vi "TAT_Start_old.vi"(8 "error In":errorcluster) -> (0 "error out":errorcluster)   [LabVIEW 2017]
uses:
  Controls/Ass. Loop Control.ctl
  <vilib>/addons/database/NI_Database_API.lvlib
  <vilib>/addons/database/Connection.llb/DB Tools Open Connec (Path).vi
  <vilib>/Instr/_visa.llb/VISA Configure Serial Port (Instr).vi
  <vilib>/addons/database/Connection.llb/Conn ObjectReference.ctl
  <vilib>/Utility/error.llb/DialogType.ctl
panel:
  out "BARCODE STATION 3":string caption="BARCODE:-"
  out "LEAK UNIT RESULT 2":bool caption="LEAK RESULT:-"
  out "LEAK ACTUAL VALUE 2":string
  out "LEAK MAX 2":string
  out "LEAK MIN 2":string
  out "LEAK UNIT RESULT":bool caption="LEAK RESULT:-"
  out "LEAK ACTUAL VALUE":string
  out "LEAK MAX":string
  out "LEAK MIN":string
  out "PREVIOUS BARCODE":string[](array[string])
  out "scanned":string
  out "PACKAGE Qty  2":string
  out "PROJECT :-":string
  out "PACKAGE Qty":string
  out "TORISHI CODE:-":string
  out "PART No.:-":string
  out "PLC COMMUNICATION":bool
  in  "Stop":bool
  out "BARCODE STATION 2":string caption="BARCODE:-"
  out "RESULT STATION 1":bool caption="FINAL RESULT:-"
  out "USER:-":string
  out "PART NAME :-":string
  in  "ASS-Alarms":bool
  out "CYCLE STATUS STATION 1":string caption="CYCLE STATUS:-"
  out "DATE/TIME":string
  # "KAPSE SONS ROBOTICS\n& AUTOMATION"
  # "PACKAGING SLIP"
  # "MODEL SELECTED"
  # "SCANNED QUANTITY"
  # "PACKAGE QUANTITY"
  # "LEAK TESTING PARAMETER"
  # "MIN"
  # "MAX"
  # "ACTUAL VALUE"
  # "RESULT"
  # "LEAK UNIT"
  # "LEAK PRESSURE"
  # "PREVIOUS BARCODE"
  # "Nm"
  # "POKA-YOKE STATUS"
  # "XBA ORVM"
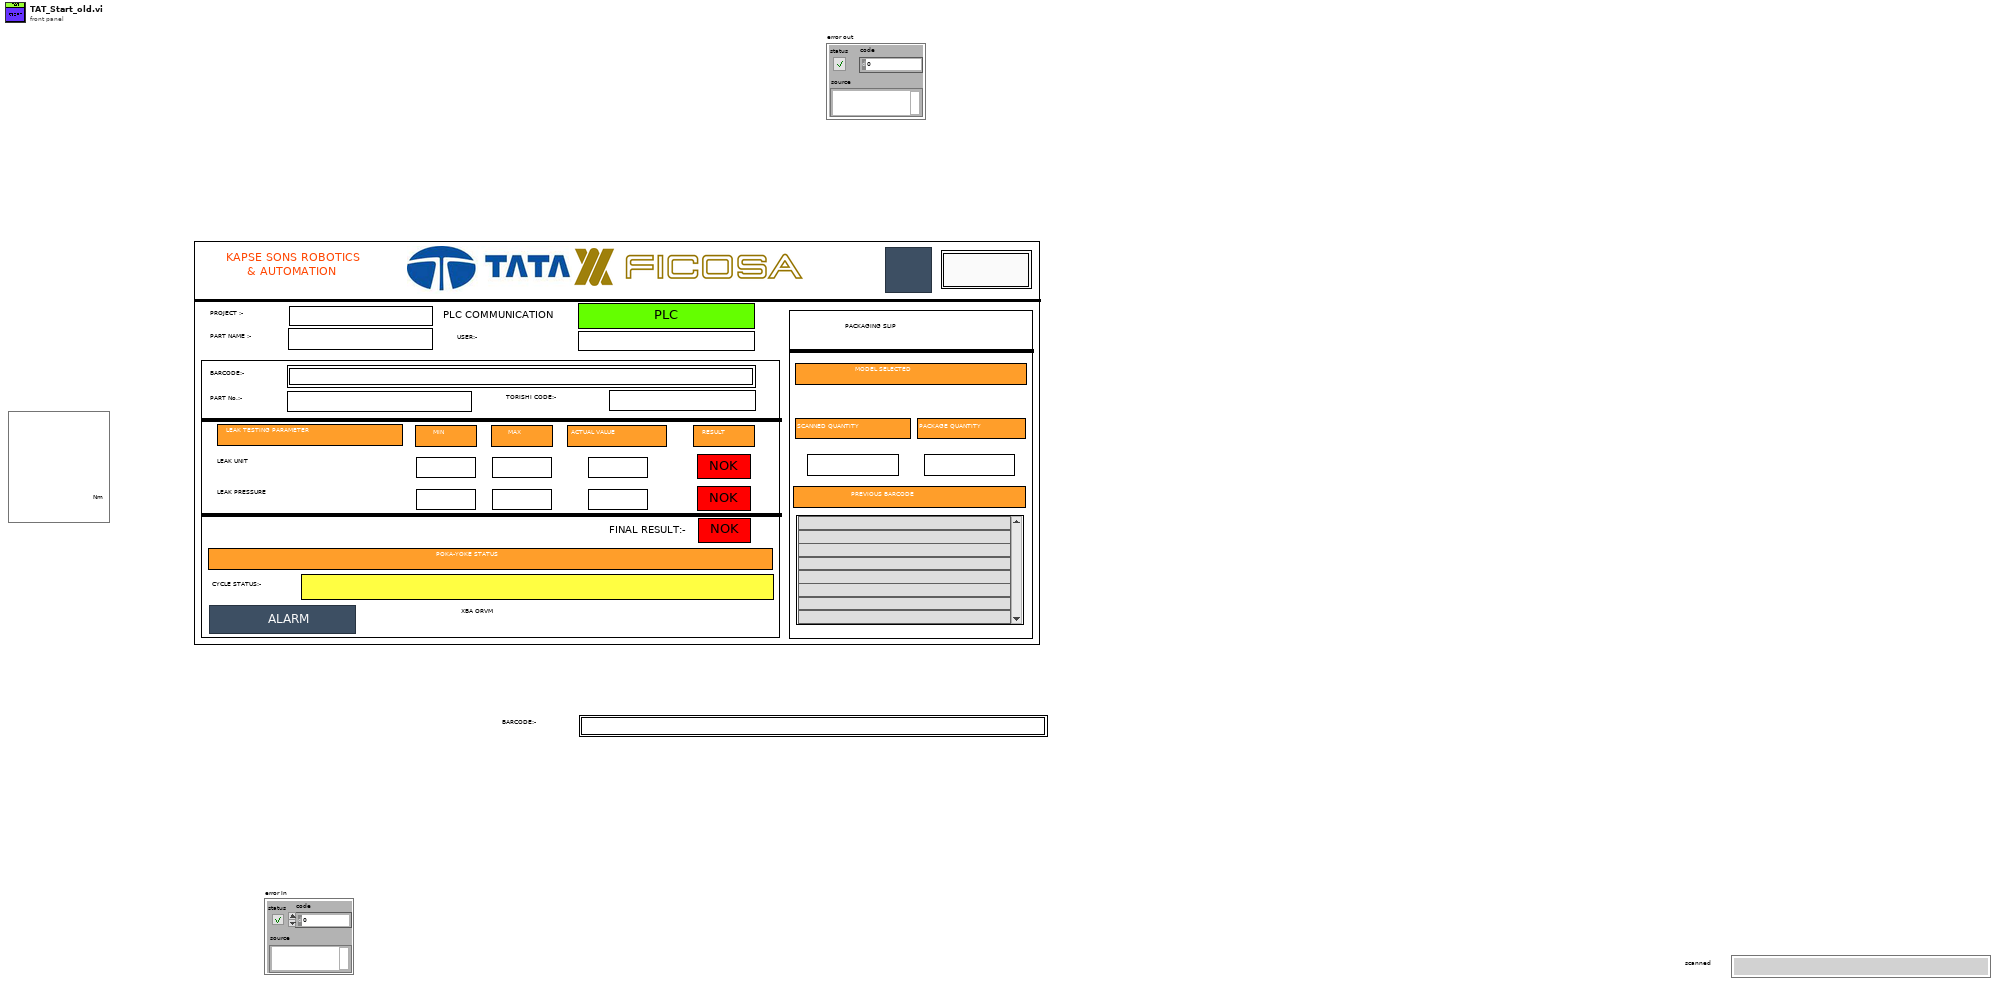
[diagram p1: front panel]
types:
  T1 = typedef "Ass. Loop Control.ctl" = enum16{"Package_Qty_Count", "GENERATE_QR_PRNT", "Cluster_update", "Waiting_for_scan", "barcode CHECK", "Int", "SaveReport ", "Barcode Print", "Start Cycle", "Wait", "Cycle End", "Stop"}
  T2 = typedef "DialogType.ctl" = u16
  T3 = typedef "NI_Database_API.lvlib/Conn ObjectReference.ctl" = refnum<k1>
  T4 = cluster{"Varient number":u16, "Part name":string, "Barcode":string, "connection reference":T3, "Batch_Size":u16, "PART_NO":string, "TORISHI_CODE":string, "printer com":refnum<visa-resource-name>, "scanner com":refnum<visa-resource-name>}
  T5 = cluster{"seconds since 1Jan1904":timestamp, "Part name":string, "BARCODE STATION 2":string, "table":string, "table":string}
  T6 = cluster{"date string":string, "time string":string, "Part name":string, "PART_NO":string, "TORISHI_CODE":string, "table":string, "table":string, string}
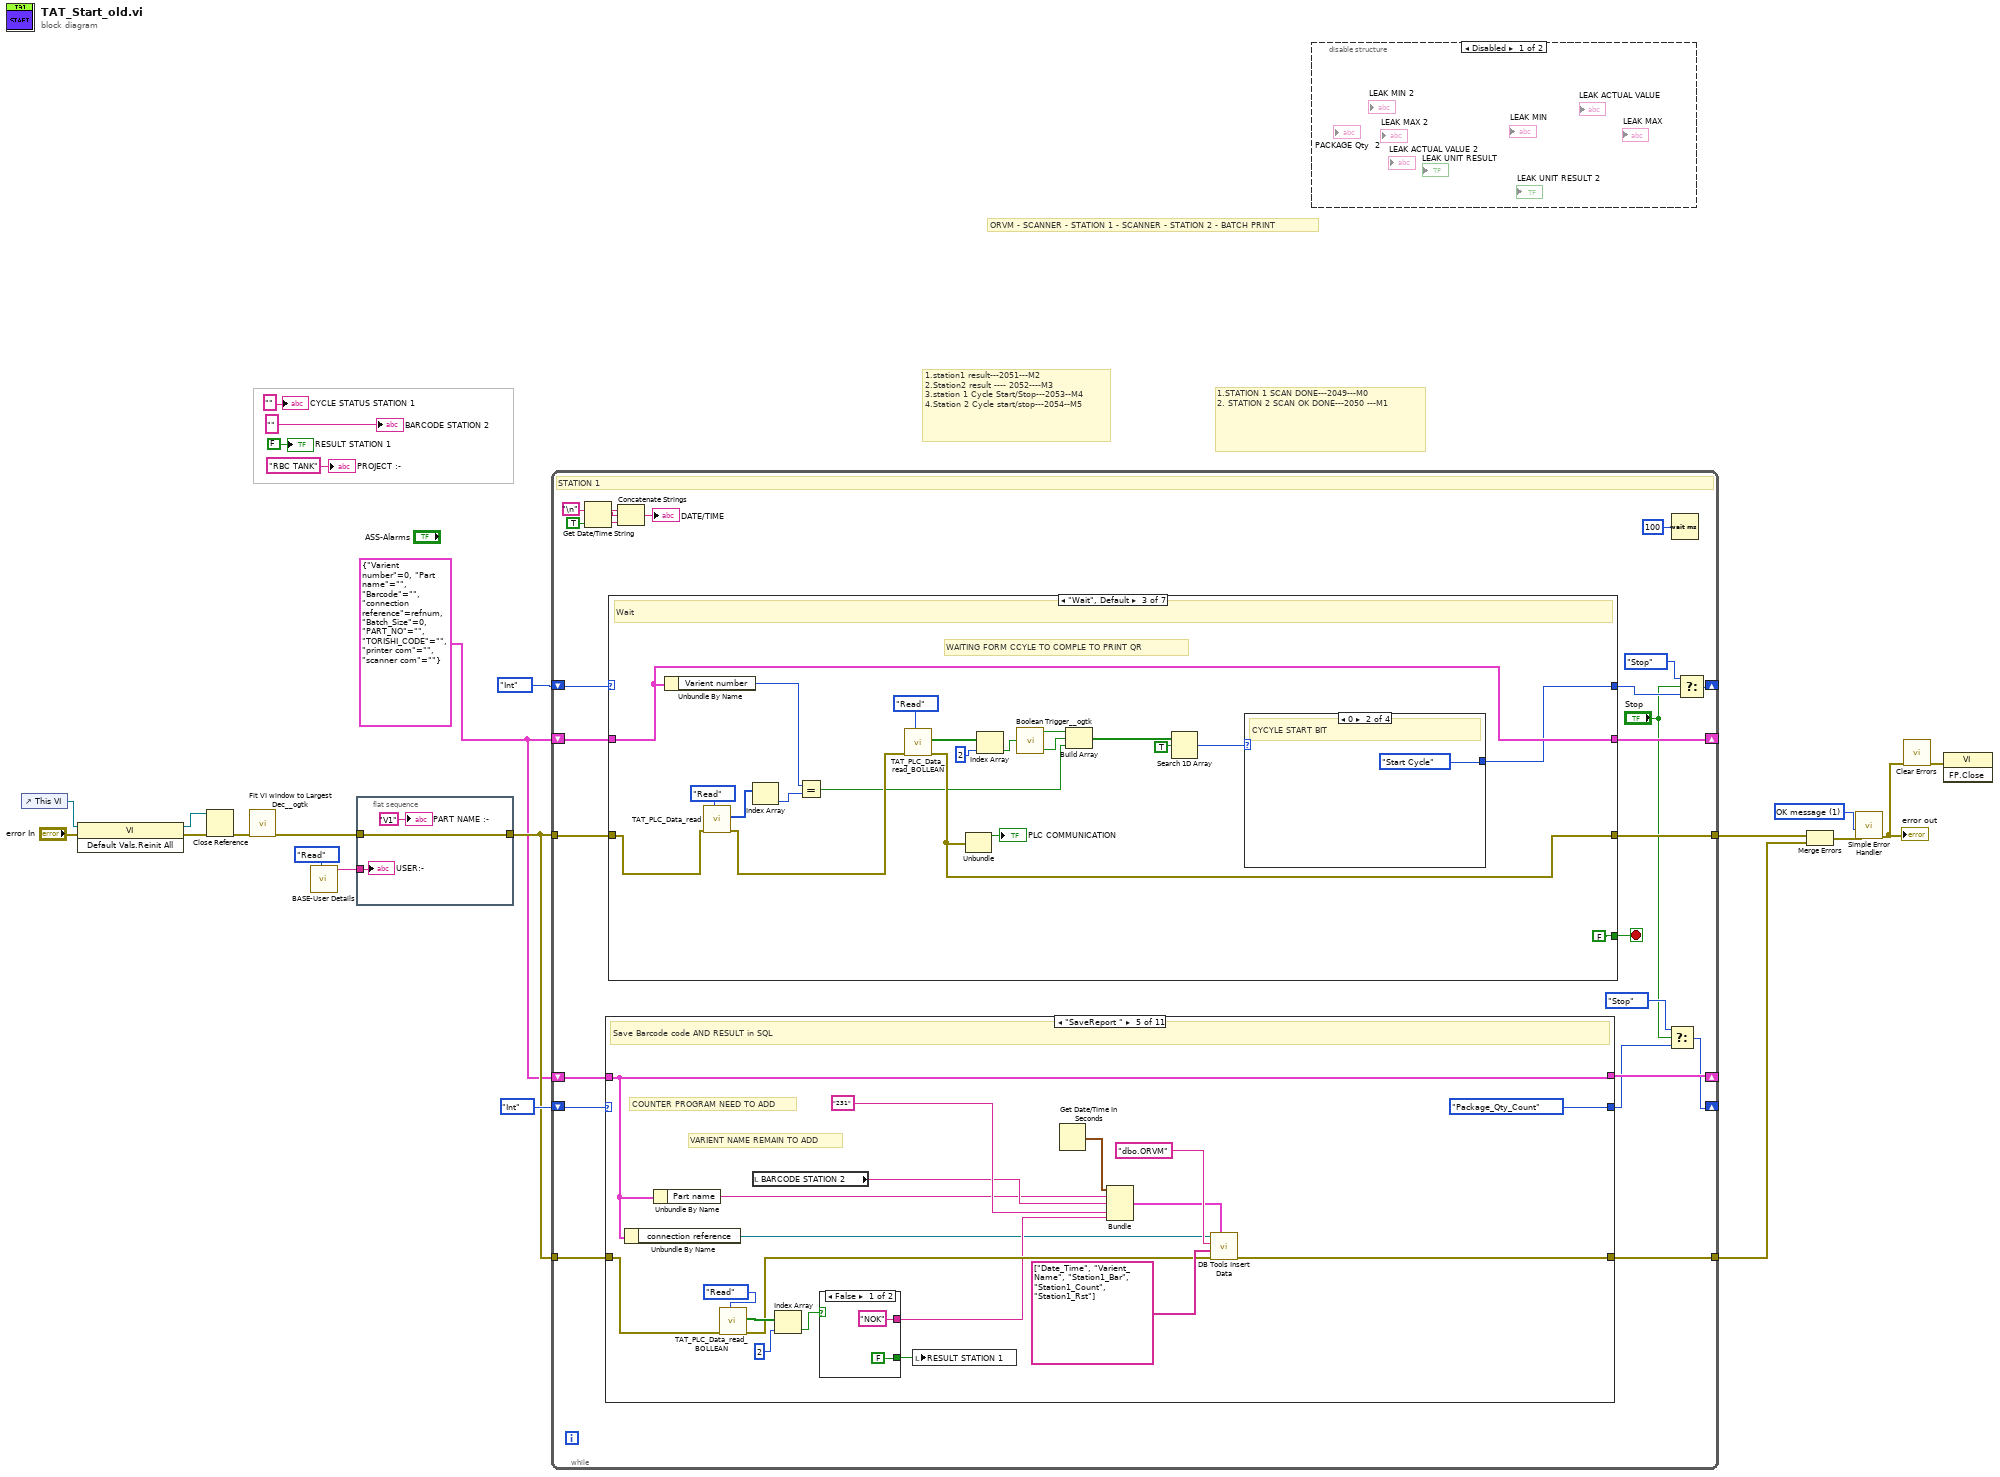
[diagram p0: block diagram]
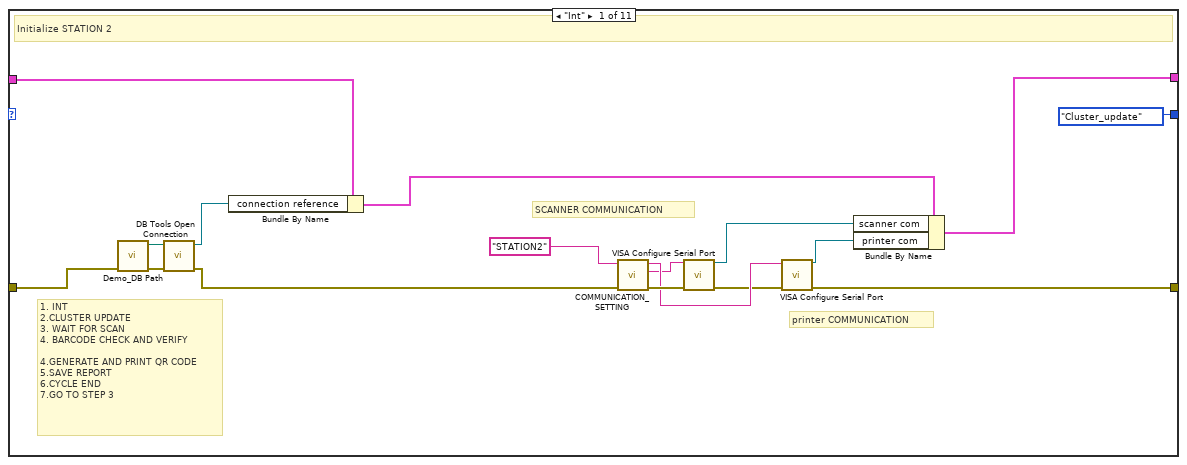
[diagram p3: hidden frame]
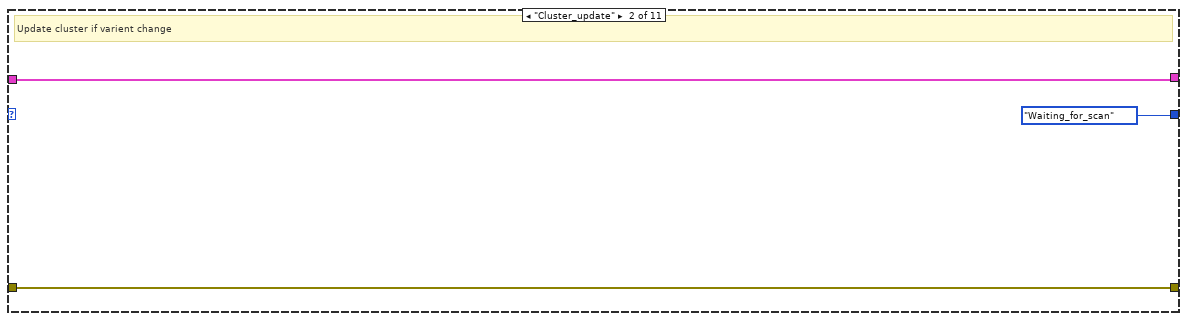
[diagram p4: hidden frame]
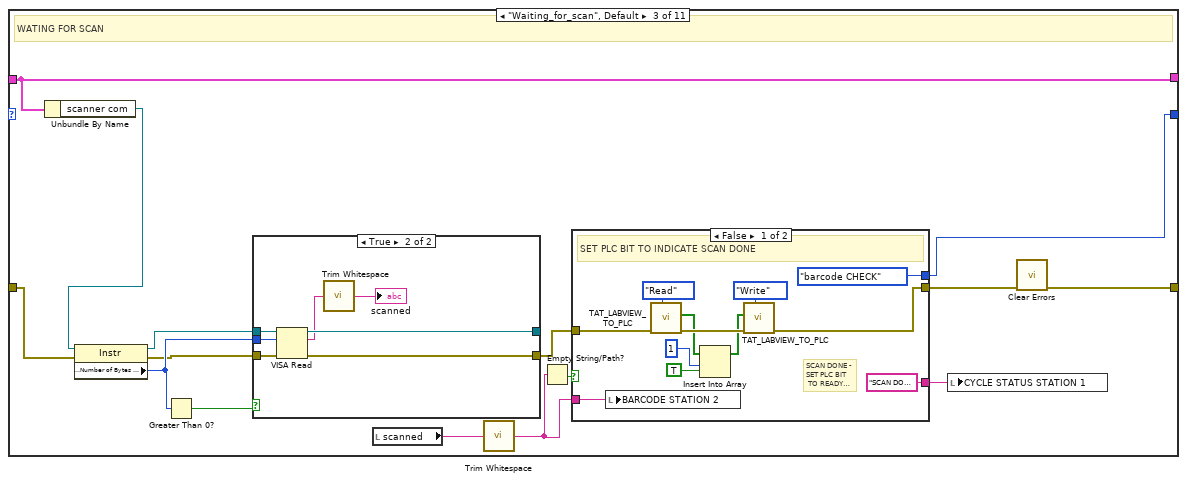
[diagram p5: hidden frame]
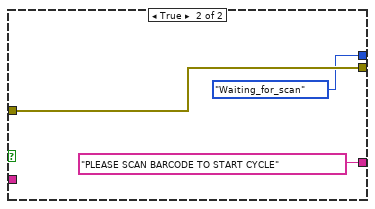
[diagram p7: hidden frame]
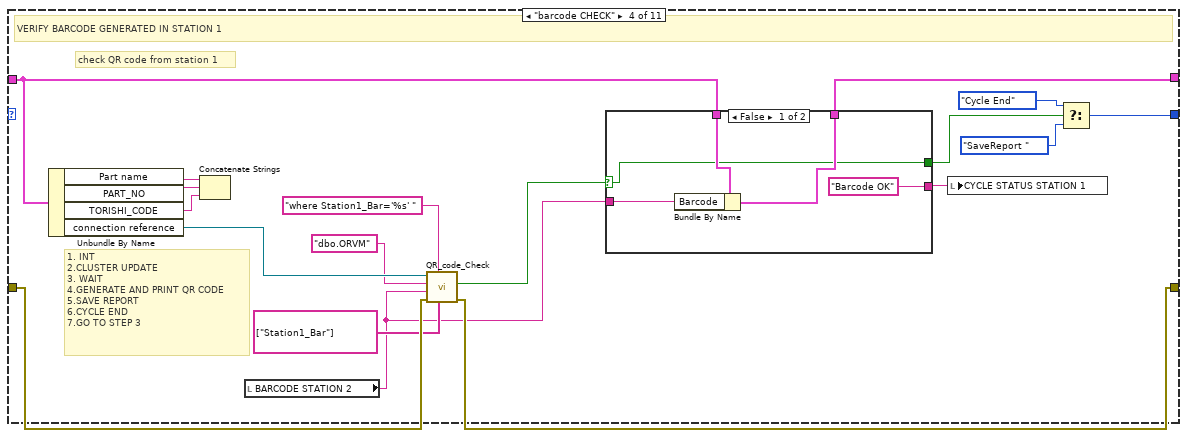
[diagram p8: hidden frame]
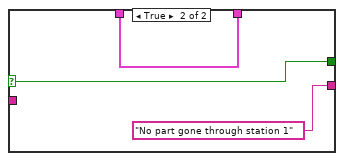
[diagram p9: hidden frame]
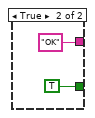
[diagram p10: hidden frame]
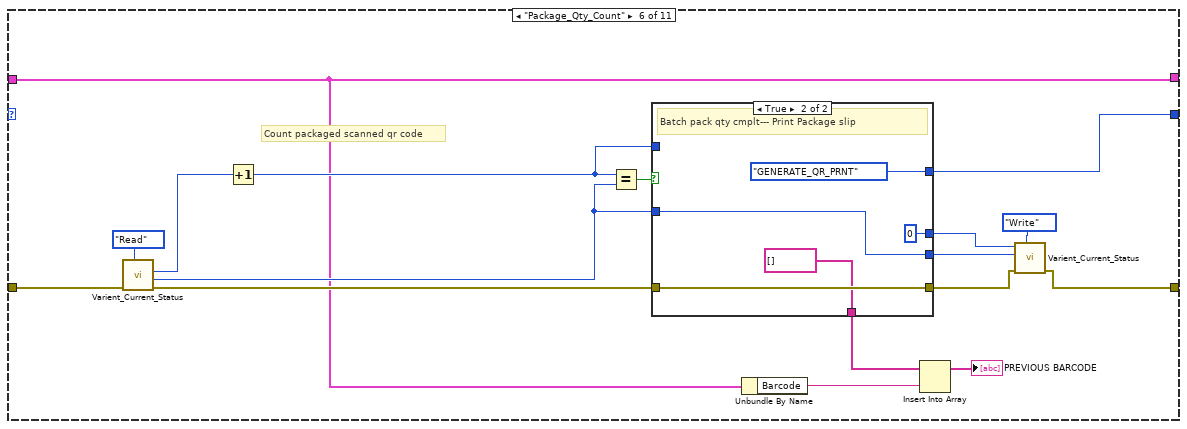
[diagram p11: hidden frame]
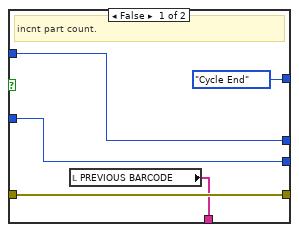
[diagram p12: hidden frame]
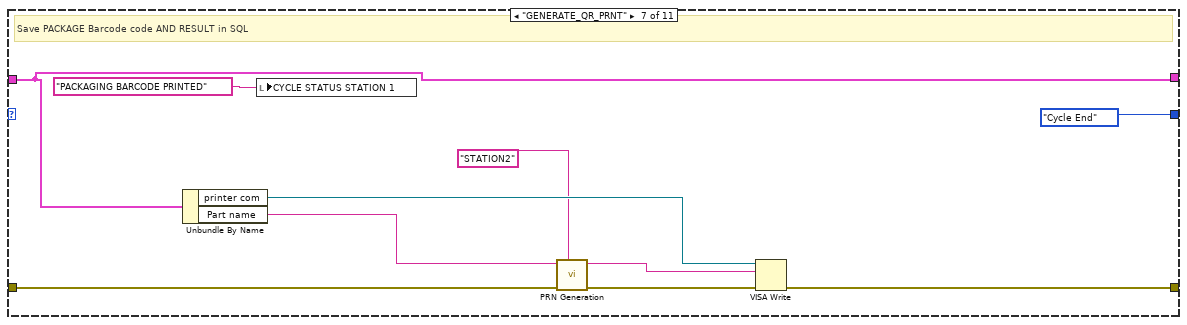
[diagram p13: hidden frame]
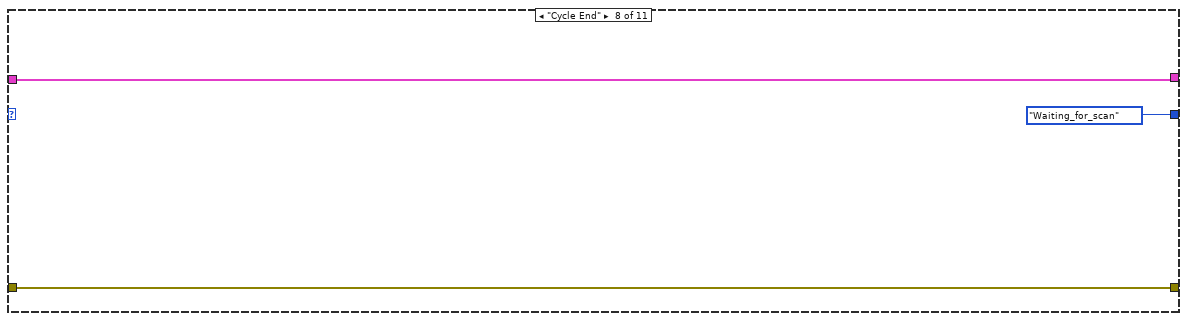
[diagram p14: hidden frame]
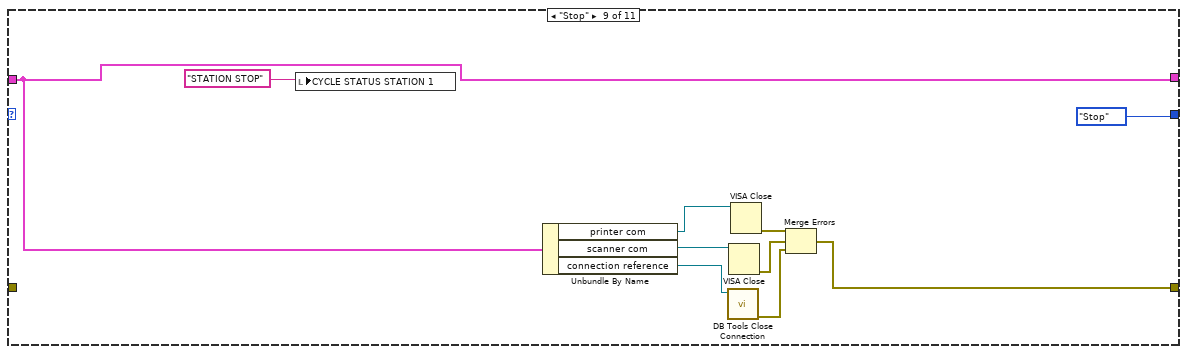
[diagram p15: hidden frame]
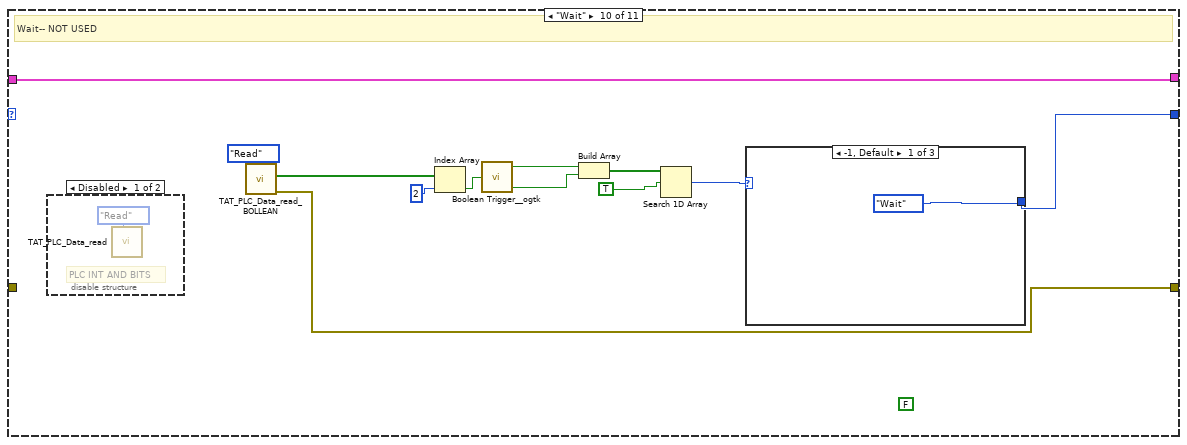
[diagram p16: hidden frame]
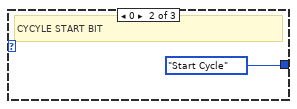
[diagram p18: hidden frame]
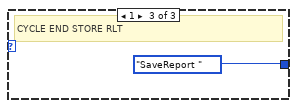
[diagram p19: hidden frame]
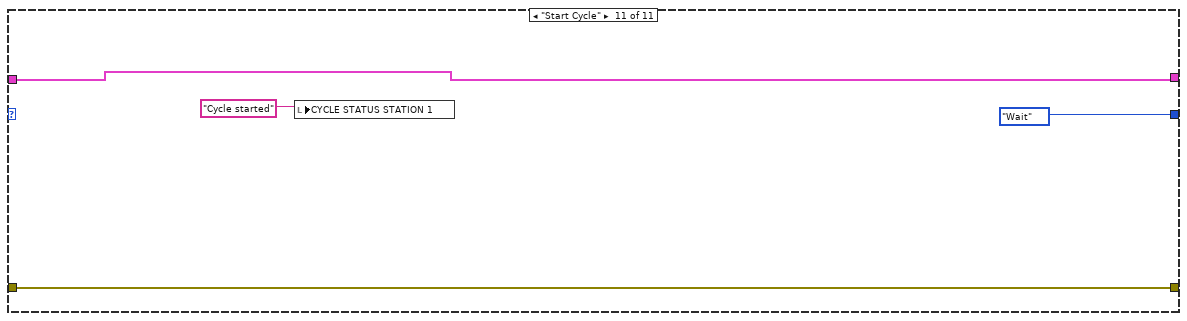
[diagram p20: hidden frame]
diagram:
  w6 = T2 1 items=["no dialog", "OK message", "continue or stop message", "OK message + warnings", "continue/stop + warnings"] ("type of dialog (OK msg:1)")
  w2 = T4 {"Varient number"=0, "Part name"="", "Barcode"="", "connection reference"=refnum, "Batch_Size"=0, "PART_NO"="", "TORISHI_CODE"="", "printer com"="", "scanner com"=""}
  # "1.STATION 1 SCAN DONE---2049---M0\n2. STATION 2 SCAN OK DONE---2050 ---M1"
  # "1.station1 result---2051---M2\n2.Station2 result ---- 2052----M3\n3.station 1 Cycle Start/Stop---2053--M4\n4.Station 2 Cycle start/stop---2054--M5"
  # "ORVM - SCANNER - STATION 1 - SCANNER - STATION 2 - BATCH PRINT"
  n1 = control-ref of="This VI"() -> (w22:refnum<vi>)
  n2 = invoke class="VI" method="Default Vals.Reinit All"(reference=w22, error in="error In") -> (reference out=w19:refnum<vi>, error out=w20:errorcluster)  [unwired: 1 in, 1 out]
  n3 = Close Reference(reference=w19, error in (no error)=w20) -> (error out=w18:errorcluster)
  n4 = call <userlib>:"Fit VI window to Largest Dec__ogtk.vi"("error in (no error)"=w18) -> ("error out"=w17:errorcluster)  [unwired: 5 in, 1 out]
  n5 = call "BASE-User Details.vi"("Enum"=enum16{"Read", "Write"}."Read") -> ("User Name Out"=w7:string)  [unwired: 9 in, 1 out]
  n6 = flat-sequence {
    tunnel: [w25] -> w3
    tunnel: w17 -> [w25]
    tunnel: w7 -> [w23]
    frame #0 {
      "USER:-" <- w23
      "PART NAME :-" <- "V1"
    }
  }
  n7 = while {
    tunnel: w3 -> [w44]
    shift-right: [w43] -> _
    shift-left: Ass._Loop_Control."Int" ("Enum") -> [w49]
    shift-right: [w47] -> _
    shift-left: w2 -> [w46]
    tunnel: [w45] -> w13
    shift-right: [w28] -> _
    shift-left: Ass._Loop_Control."Int" ("Enum") -> [w34]
    tunnel: w3 -> [w33]
    shift-right: [w31] -> _
    shift-left: w2 -> [w32]
    tunnel: [w30] -> w1
    stop <- w35 stop-if-true
    # "STATION 1"
    n8 = Get Date/Time String(want seconds? (F)=TRUE) -> (date string=w39:string, time string=w38:string)  [unwired: 2 in]
    n9 = case shown="\"SaveReport \"" w34 {
      tunnel: [Ass._Loop_Control."Cluster_update" ("Enum") Ass._Loop_Control."Waiting_for_scan" ("Enum") w72 w126 Ass._Loop_Control."Package_Qty_Count" ("Enum") w162 Ass._Loop_Control."Cycle End" ("Enum") Ass._Loop_Control."Waiting_for_scan" ("Enum") Ass._Loop_Control."Stop" ("Enum") w214 Ass._Loop_Control."Wait" ("Enum")] -> w27
      tunnel: [w63 w67 w71 w120 w137 w159 w189 w195 w201 w208 w224] -> w31
      tunnel: [w62 w68 w82 w118 w136 w168 w190 w196 w203 w210 w225] -> w30
      tunnel: w33 -> [w51 w68 w75 w119 w135 w174 w186 w196 _ _ w225]
      tunnel: w32 -> [w50 w67 w71 w121 w137 w159 w189 w195 w201 w208 w224]
      frame "Int" {
        # "1. INT\n2.CLUSTER UPDATE\n3. WAIT FOR SCAN\n4. BARCODE CHECK AND VERIFY\n\n4.GENERATE AND PRINT QR CODE\n5.SAVE REPORT\n6.CYCLE END\n7.GO TO STEP 3"
        # "printer COMMUNICATION"
        # "SCANNER COMMUNICATION"
        # "Initialize STATION 2"
        n10 = call "Demo_DB Path.vi"("error in"=w51) -> ("error out"=w54:errorcluster, "DB Path"=w56:path)  [unwired: 9 in]
        n11 = call-poly <vilib>:"DB Tools Open Connection.vi"("error in (no error)"=w54, "connection information"=w56) -> ("error out"=w53:errorcluster, "connection reference"=w52:T3)  [unwired: 6 in]
        n12 = Bundle By Name(cluster=w50, "connection reference"=w52) -> (w55:T4)
        n13 = call "COMMUNICATION_SETTING.vi"("error in"=w53, "STATION"="STATION2") -> ("error out"=w65:errorcluster, "SCAN_COM"=w57:string, "PRINT_COM"=w61:string)  [unwired: 7 in]
        n14 = call-poly "VISA Configure Serial Port"("VISA resource name"=w57, "error in (no error)"=w65) -> ("VISA resource name out"=w58:refnum<visa-resource-name>, "error out"=w59:errorcluster)  [unwired: 12 in]
        n15 = call-poly "VISA Configure Serial Port"("VISA resource name"=w61, "error in (no error)"=w59) -> ("VISA resource name out"=w60:refnum<visa-resource-name>, "error out"=w62:errorcluster)  [unwired: 12 in]
        n16 = Bundle By Name(cluster=w55, "scanner com"=w58, "printer com"=w60) -> (w63:T4)
      }
      frame "Cluster_update" {
        # "Update cluster if varient change"
      }
      frame "Waiting_for_scan", Default {
        # "WATING FOR SCAN"
        n17 = Unbundle By Name(w71) -> ("scanner com"=w70:refnum<visa-resource-name>)
        n18 = property class="Instr"(reference=w70, error in=w75) -> (reference out=w80:refnum<visa-resource-name>, error out=w79:errorcluster, "Serial Settings:Number of Bytes at Serial Port"=w81:u32)
        n19 = Greater Than 0?(x=w81) -> (x > 0?=w78:bool)
        n20 = case shown="True" w78 {
          tunnel: w80 -> [w86 w93]
          tunnel: w79 -> [w85 w92]
          tunnel: w81 -> [_ w91]
          tunnel: [w86 w90] -> _
          tunnel: [w85 w89] -> w77
          frame False {
          }
          frame True {
            n21 = VISA Read(VISA resource name=w93, byte count=w91, error in (no error)=w92) -> (VISA resource name out=w90:refnum<visa-resource-name>, read buffer=w88:string, error out=w89:errorcluster)  [unwired: 1 out]
            n22 = call <vilib>:"Trim Whitespace.vi"("string"=w88) -> ("trimmed string"=→"scanned":string)  [unwired: 1 in]
          }
        }
        n23 = local read "scanned"() -> (w74:string)
        n24 = call <vilib>:"Trim Whitespace.vi"("string"=w74) -> ("trimmed string"=w73:string)  [unwired: 1 in]
        n25 = Empty String/Path?(string/path=w73) -> (empty?=w84:bool)
        n26 = case shown="False" w84 {
          tunnel: ["SCAN DONE WAITING TO START CYCYLE" ("Cycle Status") "PLEASE SCAN BARCODE TO START CYCLE" ("Cycle Status")] -> w83
          tunnel: w77 -> [w101 w107]
          tunnel: [w104 w107] -> w76
          tunnel: w73 -> [w96 _]
          tunnel: [Ass._Loop_Control."barcode CHECK" ("Enum") Ass._Loop_Control."Waiting_for_scan" ("Enum")] -> w72
          frame False {
            # "SCAN DONE - SET PLC BIT\n TO READY CYCLE"
            # "SET PLC BIT TO INDICATE SCAN DONE"
            n27 = local write "BARCODE STATION 2"(w96) -> ()
            n28 = call "TAT_LABVIEW_TO_PLC.vi"("Enum"=enum16{"Read", "Write"}."Read", "error in (no error)"=w101) -> ("error out"=w100:errorcluster, "Array 2"=w99:bool[])  [unwired: 8 in]
            n29 = Insert Into Array(array=w99, index=1, new element=TRUE) -> (w98:bool[])
            n30 = call "TAT_LABVIEW_TO_PLC.vi"("Enum"=enum16{"Read", "Write"}."Write", "error in (no error)"=w100, "Array"=w98) -> ("error out"=w104:errorcluster)  [unwired: 7 in, 1 out]
          }
          frame True {
          }
        }
        n31 = local write "CYCLE STATUS STATION 1"(w83) -> ()
        n32 = call <vilib>:"Clear Errors.vi"("error in (no error)"=w76) -> ("error out"=w82:errorcluster)  [unwired: 5 in, 1 out]
      }
      frame "barcode CHECK" {
        # "check QR code from station 1"
        # "1. INT\n2.CLUSTER UPDATE\n3. WAIT\n4.GENERATE AND PRINT QR CODE\n5.SAVE REPORT\n6.CYCLE END\n7.GO TO STEP 3"
        # "VERIFY BARCODE GENERATED IN STATION 1"
        n33 = Unbundle By Name(w121) -> ("Part name"=w124:string, "PART_NO"=w123:string, "TORISHI_CODE"=w122:string, "connection reference"=w116:T3)
        n34 = Concatenate Strings(w124, w123, w122) -> ()  [unwired: 1 out]
        n35 = local read "BARCODE STATION 2"() -> (w109:string)
        n36 = call "QR_code_Check.vi"("Columns"=string[] ["Station1_Bar"] ("columns 2"), "format string"="where Station1_Bar='%s' ", "error in (no error)"=w119, "replace %s"=w109, "table"="dbo.ORVM", "Refnum in"=w116) -> ("error out"=w118:errorcluster, "ON no barcode NOT PRESENT"=w113:bool)  [unwired: 3 in, 1 out]
        n37 = case shown="False" w113 {
          selector: w113 -> [w127 w132]
          tunnel: ["Barcode OK" ("Cycle Status") "No part gone through station 1" ("Cycle Status")] -> w125
          tunnel: w121 -> [w130 w133]
          tunnel: [w129 w133] -> w120
          tunnel: w109 -> [w128 _]
          tunnel: [w127 w132] -> w110
          frame False {
            n38 = Bundle By Name(cluster=w130, "Barcode"=w128) -> (w129:T4)
          }
          frame True {
          }
        }
        n39 = local write "CYCLE STATUS STATION 1"(w125) -> ()
        n40 = Select(t=Ass._Loop_Control."Cycle End" ("Enum"), s=w110, f=Ass._Loop_Control."SaveReport " ("Enum")) -> (s? t:f=w126:T1)
      }
      frame "SaveReport " {
        # "COUNTER PROGRAM NEED TO ADD"
        # "VARIENT NAME REMAIN TO ADD"
        # "Save Barcode code AND RESULT in SQL"
        n41 = Unbundle By Name(w137) -> ("connection reference"=w138:T3)
        n42 = Unbundle By Name(w137) -> ("Part name"=w146:string)
        n43 = call "TAT_PLC_Data_read_BOLLEAN.vi"("Enum"=enum16{"Read", "Write"}."Read", "error in (no error)"=w135) -> ("error out"=w143:errorcluster, "Array 2"=w144:bool[])  [unwired: 8 in]
        n44 = local read "BARCODE STATION 2"() -> (w147:string)
        n45 = Index Array(array=w144, index=2) -> (element=w140:bool)
        n46 = case shown="False" w140 {
          tunnel: ["NOK" ("table") "OK" ("table")] -> w141
          tunnel: [FALSE TRUE] -> w139
          frame False {
          }
          frame True {
          }
        }
        n47 = local write "RESULT STATION 1"(w139) -> ()
        n48 = Get Date/Time In Seconds() -> (seconds since 1Jan1904=w148:timestamp)
        n49 = Bundle("seconds since 1Jan1904"=w148, "Part name"=w146, "BARCODE STATION 2"=w147, "table"="231", "table"=w141) -> (w151:T5)  [unwired: 1 in]
        n50 = call <vilib>:"DB Tools Insert Data.vi"("data"=w151, "error in (no error)"=w143, "columns"=string[] ["Date_Time", "Varient_Name", "Station1_Bar", "Station1_Count", "Station1_Rst"] ("columns 2"), "table"="dbo.ORVM", "connection reference"=w138) -> ("error out"=w136:errorcluster)  [unwired: 5 in, 1 out]
      }
      frame "Package_Qty_Count" {
        # "Count packaged scanned qr code"
        n51 = call "Varient_Current_Status.vi"("Enum"=enum16{"Write", "Read"}."Read", "error in"=w174) -> ("error out"=w172:errorcluster, "Batch Size"=w165:i32, "Varient Count"=w171:i32)  [unwired: 7 in]
        n52 = Increment(x=w171) -> (x+1=w166:i32)
        n53 = Equal?(x=w166, y=w165) -> (x = y?=w170:bool)
        n54 = case shown="True" w170 {
          tunnel: [w179 w184] -> w167
          tunnel: w172 -> [w179 w184]
          tunnel: w166 -> [w177 _]
          tunnel: w165 -> [w178 w183]
          tunnel: [w178 w183] -> w164
          tunnel: [w177 0] -> w163
          tunnel: [Ass._Loop_Control."Cycle End" ("Enum") Ass._Loop_Control."GENERATE_QR_PRNT" ("Enum")] -> w162
          tunnel: [w175 string[] [] ("PREVIOUS BARCODE")] -> w160
          frame False {
            # "incnt part count."
            n55 = local read "PREVIOUS BARCODE"() -> (w175:string[])
          }
          frame True {
            # "Batch pack qty cmplt--- Print Package slip"
          }
        }
        n56 = Unbundle By Name(w159) -> ("Barcode"=w158:string)
        n57 = Insert Into Array(array=w160, new element=w158) -> (→"PREVIOUS BARCODE":string[])  [unwired: 1 in]
        n58 = call "Varient_Current_Status.vi"("Enum"=enum16{"Write", "Read"}."Write", "error in"=w167, "Batch Size"=w164, "Varient count"=w163) -> ("error out"=w168:errorcluster)  [unwired: 5 in, 2 out]
      }
      frame "GENERATE_QR_PRNT" {
        # "Save PACKAGE Barcode code AND RESULT in SQL"
        n59 = Unbundle By Name(w189) -> ("printer com"=w188:refnum<visa-resource-name>, "Part name"=w187:string)
        n60 = local write "CYCLE STATUS STATION 1"("PACKAGING BARCODE PRINTED" ("Cycle Status")) -> ()
        n61 = call "PRN Generation.vi"(7:"STATION2" ("FILE NAME"), "error in (no error)"=w186, 11:w187) -> ("error out"=w192:errorcluster, "PRN to Print"=w191:string)  [unwired: 6 in, 1 out]
        n62 = VISA Write(VISA resource name=w188, write buffer=w191, error in (no error)=w192) -> (error out=w190:errorcluster)  [unwired: 2 out]
      }
      frame "Cycle End" {
      }
      frame "Stop" {
        n63 = local write "CYCLE STATUS STATION 1"("STATION STOP" ("Cycle Status")) -> ()
        n64 = Unbundle By Name(w201) -> ("printer com"=w200:refnum<visa-resource-name>, "scanner com"=w199:refnum<visa-resource-name>, "connection reference"=w198:T3)
        n65 = call <vilib>:"DB Tools Close Connection.vi"("connection reference"=w198) -> ("error out"=w202:errorcluster)  [unwired: 6 in]
        n66 = VISA Close(VISA resource name=w199) -> (error out=w204:errorcluster)  [unwired: 1 in]
        n67 = VISA Close(VISA resource name=w200) -> (error out=w205:errorcluster)  [unwired: 1 in]
        n68 = Merge Errors(w205, w204, w202) -> (w203:errorcluster)
      }
      frame "Wait" {
        (unwired) FALSE
        # "Wait-- NOT USED"
        n69 = disable-structure shown="Disabled" {
          frame Disabled {
            # "PLC INT AND BITS"
            n70 = call "TAT_PLC_Data_read.vi"("Enum"=enum16{"Read", "Write"}."Read") -> ()  [unwired: 9 in, 2 out]
          }
          frame Enabled {
          }
        }
        n71 = call "TAT_PLC_Data_read_BOLLEAN.vi"("Enum"=enum16{"Read", "Write"}."Read") -> ("error out"=w210:errorcluster, "Array 2"=w211:bool[])  [unwired: 9 in]
        n72 = Index Array(array=w211, index=2) -> (element=w212:bool)
        n73 = call <userlib>:"Boolean Trigger__ogtk.vi"("Boolean Input"=w212) -> ("Rising Edge"=w218:bool, "Falling Edge"=w216:bool)  [unwired: 1 in]
        n74 = Build Array(w218, w216) -> (w217:bool[])
        n75 = Search 1D Array(1D array=w217, element=TRUE ("Boolean Input")) -> (index of element=w215:i32)  [unwired: 1 in]
        n76 = case shown="-1, Default" w215 {
          tunnel: [Ass._Loop_Control."Wait" ("Enum") Ass._Loop_Control."Start Cycle" ("Enum") Ass._Loop_Control."SaveReport " ("Enum")] -> w214
          frame -1, Default {
          }
          frame 0 {
            # "CYCYLE START BIT"
          }
          frame 1 {
            # "CYCLE END STORE RLT"
          }
        }
      }
      frame "Start Cycle" {
        n77 = local write "CYCLE STATUS STATION 1"("Cycle started" ("Cycle Status")) -> ()
      }
    }
    n78 = case shown="\"Wait\", Default" w49 {
      tunnel: [Ass._Loop_Control."Cluster_update" ("Enum") Ass._Loop_Control."Wait" ("Enum") w256 Ass._Loop_Control."Wait" ("Enum") Ass._Loop_Control."Cycle End" ("Enum") Ass._Loop_Control."Wait" ("Enum") Ass._Loop_Control."Stop" ("Enum")] -> w42
      tunnel: [w232 w248 w258 w283 w295 w315 w320] -> w47
      tunnel: w46 -> [w233 w249 w258 w283 w295 w315 w320]
      tunnel: [_ _ FALSE _ _ _ TRUE] -> w35
      tunnel: [w229 w239 w265 w280 w305 w314 w317] -> w45
      tunnel: w44 -> [w230 w251 w260 w280 w297 w314 w318]
      frame "Int" {
        # "1. INT\n2.CLUSTER UPDATE\n3. WAIT\n4.\n5.SAVE REPORT\n6.CYCLE END\n7.GO TO STEP 3"
        # "Initialize"
        n79 = call "Demo_DB Path.vi"("error in"=w230) -> ("error out"=w231:errorcluster, "DB Path"=w234:path)  [unwired: 9 in]
        n80 = call-poly <vilib>:"DB Tools Open Connection.vi"("error in (no error)"=w231, "connection information"=w234) -> ("error out"=w229:errorcluster, "connection reference"=w228:T3)  [unwired: 6 in]
        n81 = local write "CYCLE STATUS STATION 1"("WAIT FOR CYCLE START" ("Cycle Status")) -> ()
        n82 = Bundle By Name(cluster=w233, "connection reference"=w228) -> (w232:T4)
      }
      frame "Cluster_update" {
        # "PART NAME\nPART No.\nPACKAGE QUANTITY\nTORISHI CODE"
        # "PART NAME---\nVARIENT NAME"
        # "Update cluster if varient change"
        n83 = call "TAT_PLC_Data_read.vi"("Enum"=enum16{"Read", "Write"}."Read", "error in (no error)"=w251) -> ("error out"=w242:errorcluster, "Array 2"=w253:u16[])  [unwired: 8 in]
        n84 = Index Array(array=w253) -> (element=w243:u16)  [unwired: 1 in]
        n85 = call "Varient_number_check.vi"("error in"=w242, "Varient No."=w243) -> ("error out"=w240:errorcluster, "Batch Size"=w238:i32, "Varient Number"=w250:i32, "Part Name"=w247:string, "PART_NO"=w244:string, "TORISHI_CODE"=w245:string)  [unwired: 4 in]
        "PART No.:-" <- w244
        "TORISHI CODE:-" <- w245
        n86 = Number To Decimal String(number=w238) -> (decimal integer string=→"PACKAGE Qty":string)  [unwired: 1 in]
        n87 = local write "PART NAME :-"(w247) -> ()
        n88 = Bundle By Name(cluster=w249, "Part name"=w247, "Varient number"=w250, "Batch_Size"=w238, "PART_NO"=w244, "TORISHI_CODE"=w245) -> (w248:T4)
        n89 = call "Varient_Current_Status.vi"("Enum"=enum16{"Write", "Read"}."Write", "error in"=w240, "Batch Size"=w238, "Varient count"=0) -> ("error out"=w239:errorcluster)  [unwired: 5 in, 2 out]
      }
      frame "Wait", Default {
        # "WAITING FORM CCYLE TO COMPLE TO PRINT QR"
        # "Wait"
        n90 = Unbundle By Name(w258) -> ("Varient number"=w257:u16)
        n91 = call "TAT_PLC_Data_read.vi"("Enum"=enum16{"Read", "Write"}."Read", "error in (no error)"=w260) -> ("error out"=w259:errorcluster, "Array 2"=w261:u16[])  [unwired: 8 in]
        n92 = Index Array(array=w261) -> (element=w263:u16)  [unwired: 1 in]
        n93 = Equal?(x=w257, y=w263) -> (x = y?=w255:bool)
        n94 = call "TAT_PLC_Data_read_BOLLEAN.vi"("Enum"=enum16{"Read", "Write"}."Read", "error in (no error)"=w259) -> ("error out"=w265:errorcluster, "Array 2"=w267:bool[])  [unwired: 8 in]
        n95 = Unbundle(w265) -> ("status"=→"PLC COMMUNICATION":bool)  [unwired: 2 out]
        n96 = Index Array(array=w267, index=2) -> (element=w268:bool)
        n97 = call <userlib>:"Boolean Trigger__ogtk.vi"("Boolean Input"=w268) -> ("Rising Edge"=w274:bool, "Falling Edge"=w272:bool)  [unwired: 1 in]
        n98 = Build Array(w274, w272, w255) -> (w273:bool[])
        n99 = Search 1D Array(1D array=w273, element=TRUE ("Boolean Input")) -> (index of element=w271:i32)  [unwired: 1 in]
        n100 = case shown="0" w271 {
          tunnel: [Ass._Loop_Control."Wait" ("Enum") Ass._Loop_Control."Start Cycle" ("Enum") Ass._Loop_Control."SaveReport " ("Enum") Ass._Loop_Control."Cluster_update" ("Enum")] -> w256
          frame -1, Default {
          }
          frame 0 {
            # "CYCYLE START BIT"
          }
          frame 1 {
            # "CYCLE END STORE RLT"
          }
          frame 2 {
            # "CLUSTER UPDATE"
          }
        }
      }
      frame "Start Cycle" {
        n101 = local write "CYCLE STATUS STATION 1"("Cycle started" ("Cycle Status")) -> ()
      }
      frame "SaveReport " {
        (unwired) string[] ["Date", "Time", "Part_Name", "Part_No", "Torishi_Code", "Shift", "Station1_Rst", "Packaging_Qty", "Serial_No", "QR_Code", "Station2_Rst"] ("columns 2")
        # "Save Barcode code AND RESULT in SQL"
        n102 = Unbundle By Name(w295) -> ("connection reference"=w304:T3)
        n103 = Unbundle By Name(w295) -> ("Part name"=w303:string, "PART_NO"=w291:string, "TORISHI_CODE"=w290:string, "Batch_Size"=w287:u16)
        n104 = call "TAT_PLC_Data_read_BOLLEAN.vi"("Enum"=enum16{"Read", "Write"}."Read", "error in (no error)"=w297) -> ("error out"=w300:errorcluster, "Array 2"=w301:bool[])  [unwired: 8 in]
        n105 = Number To Decimal String(number=w287) -> (decimal integer string=w286:string)  [unwired: 1 in]
        n106 = Index Array(array=w301, index=2) -> (element=w298:bool)
        n107 = case shown="False" w298 {
          tunnel: ["NOK" ("table") "OK" ("table")] -> w289
          tunnel: [FALSE TRUE] -> w296
          frame False {
          }
          frame True {
          }
        }
        n108 = local write "RESULT STATION 1"(w296) -> ()
        n109 = Get Date/Time In Seconds() -> (seconds since 1Jan1904=w294:timestamp)
        n110 = Get Date/Time String(seconds (now)=w294) -> (date string=w293:string, time string=w292:string)  [unwired: 2 in]
        n111 = Bundle("date string"=w293, "time string"=w292, "Part name"=w303, "PART_NO"=w291, "TORISHI_CODE"=w290, "table"="SHIFT TO ADD HERE", "table"=w289, w286) -> (w306:T6)  [unwired: 1 in]
        n112 = call <vilib>:"DB Tools Insert Data.vi"("data"=w306, "error in (no error)"=w300, "columns"=string[] ["Date", "Time", "Part_Name", "Part_No", "Torishi_Code", "Shift", "Station1_Rst", "Packaging_Qty"] ("columns 2"), "table"="dbo.XBA_ORVM", "connection reference"=w304) -> ("error out"=w305:errorcluster)  [unwired: 5 in, 1 out]
        n113 = local read "BARCODE STATION 2"() -> (→"BARCODE STATION 3":string)
      }
      frame "Cycle End" {
      }
      frame "Stop" {
        n114 = local write "CYCLE STATUS STATION 1"("STATION STOP" ("Cycle Status")) -> ()
        n115 = Unbundle By Name(w320) -> ("connection reference"=w316:T3)
        n116 = call <vilib>:"DB Tools Close Connection.vi"("error in (no error)"=w318, "connection reference"=w316) -> ("error out"=w317:errorcluster)  [unwired: 5 in]
      }
    }
    n117 = Concatenate Strings(w39, "\n", w38) -> (→"DATE/TIME":string)
    n118 = Select(t=Ass._Loop_Control."Stop" ("Enum"), s="Stop", f=w27) -> (s? t:f=w28:T1)
    n119 = Wait (ms)(milliseconds to wait=u32 100) -> ()  [unwired: 1 out]
    n120 = Select(t=Ass._Loop_Control."Stop" ("Enum"), s="Stop", f=w42) -> (s? t:f=w43:T1)
  }
  n121 = disable-structure shown="Disabled" {
    frame Disabled {
    }
    frame Enabled {
    }
  }
  n122 = Merge Errors(w13, w1) -> (w11:errorcluster)
  n123 = call <vilib>:"Simple Error Handler.vi"("type of dialog (OK msg:1)"=w6, "error in (no error)"=w11) -> ("error out"=w10:errorcluster)  [unwired: 3 in, 4 out]
  "error out" <- w10
  n124 = call <vilib>:"Clear Errors.vi"("error in (no error)"=w10) -> ("error out"=w9:errorcluster)  [unwired: 5 in, 1 out]
  n125 = invoke class="VI" method="FP.Close"(error in=w9) -> ()  [unwired: 2 in, 3 out]
  "CYCLE STATUS STATION 1" <- ""
  "BARCODE STATION 2" <- ""
  "RESULT STATION 1" <- FALSE ("want seconds? (F)")
  "PROJECT :-" <- "RBC TANK" ("PROJECT")
